vi "Chris_DAQ_100PSI.vi"() -> ()   [LabVIEW 2015]
uses:
  <vilib>/DAQmx/read.llb/DAQmx Read (Analog DBL 1Chan 1Samp).vi
  <vilib>/Instr/_visa.llb/VISA Configure Serial Port (Instr).vi
  <vilib>/DAQmx/create/channels.llb/DAQmx Create Channel (AI-Voltage-Basic).vi
  <vilib>/DAQmx/miscellaneous.llb/DAQmx Fill In Error Info.vi
panel:
  out "x/y":dbl
  in  "milliseconds to wait":u32
  out "Elapsed Time (s)":dbl
  out "time string":string
  in  "physical channels":tag
  out "Inlet Pressure":dbl format="%.1f"
  out "Average Flux":dbl(graph)
  out "Average Pressure":dbl(graph)
  in  "Rolling Average Length (Pressure)":u16=25
  out "Status:":bool caption="2017-05-22 4:50 PM"
  in  "Debug":bool=TRUE
  out "Aquired Data (Real Time)":cluster{"Scalar":dbl, "Filtered Volume":dbl}(graph)
  in  "Stop":bool
  out "Filtered Volume":dbl format="%.2g"
  in  "Save Path":path
  in  "Data Preview":i32(listbox)
  in  "Rolling Average Length (Flux)":u16=100
  in  "Membrane Area (sq. mm)":dbl
  in  "NI USB DAQ":tag="cDAQ2Mod1"
  in  "Filtrate Density":dbl=0.05
  in  "Flag":bool=TRUE
  in  "Precision Balance Port":refnum<visa-resource-name>="COM4"
  # "Liquid-Gated Membrane"
  # "Real-Time Data Acquisition System"
  # "Started:"
  # "Setup"
  # "COM Settings"
  # "Last Measurement:"
  # "Elapsed Time (s):"
  # "Measurement Settings"
  # "Last Updated: May 2017 • Chris Williams"
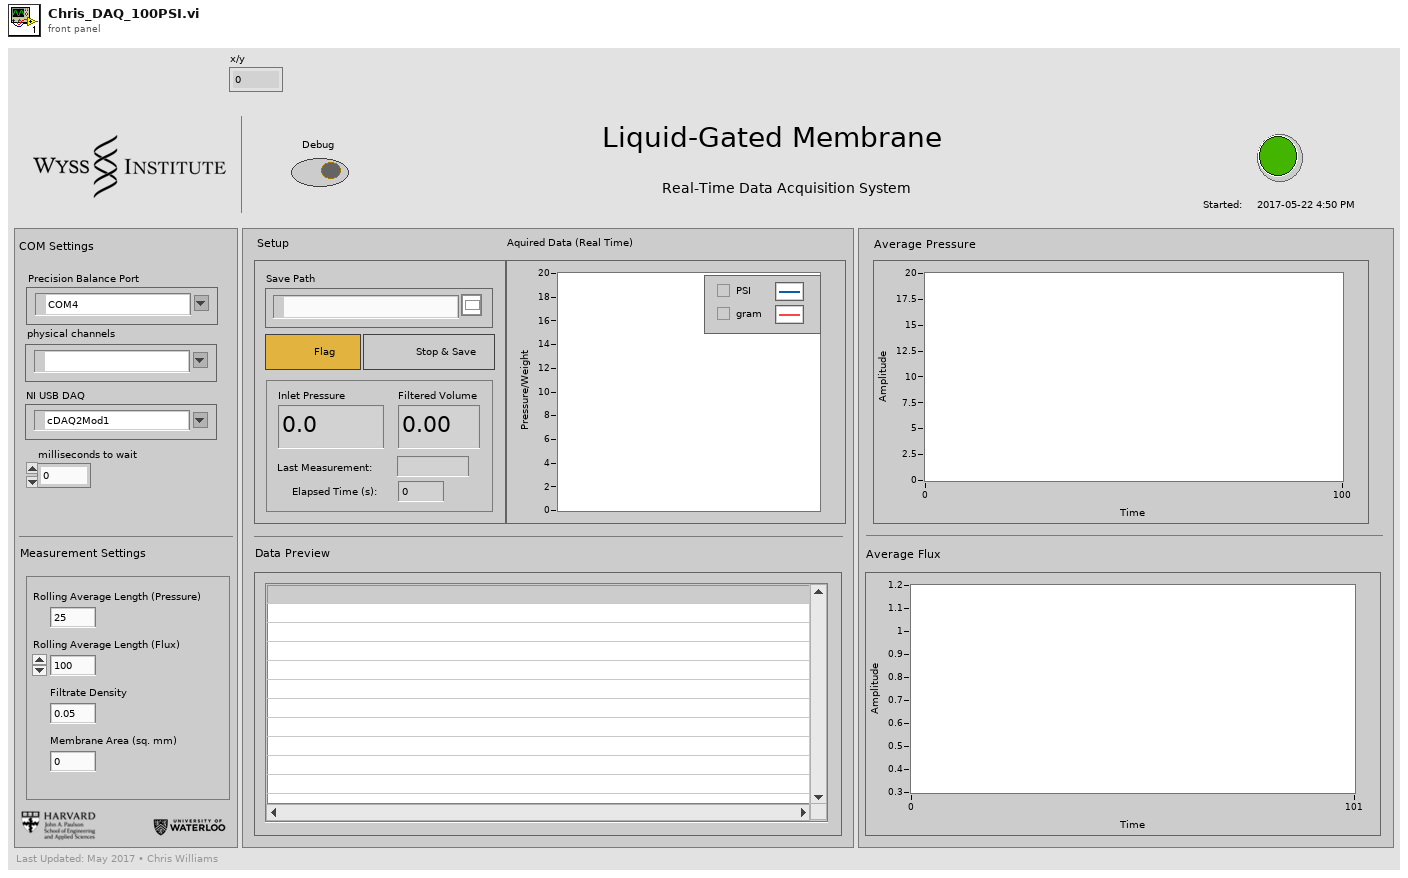
[diagram p1: front panel]
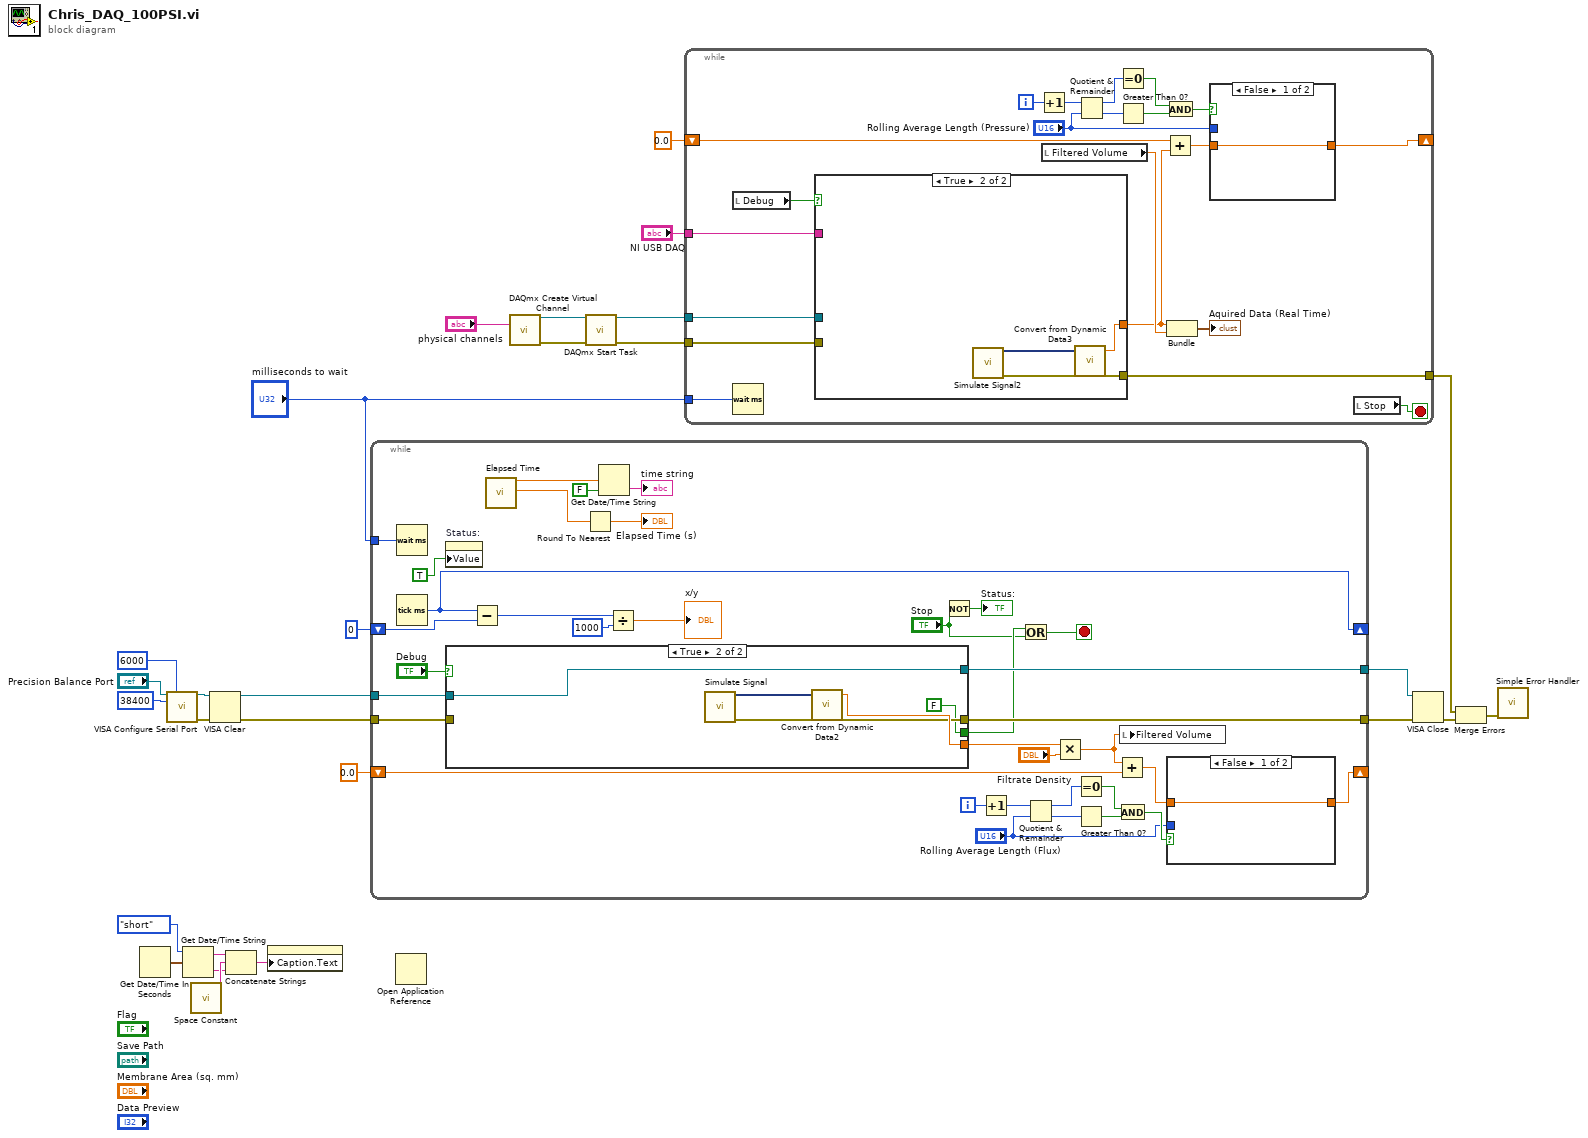
[diagram p0: block diagram]
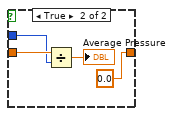
[diagram p2: hidden frame]
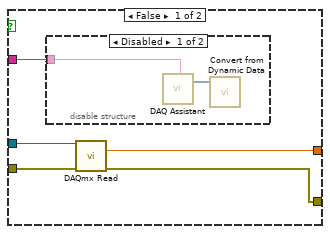
[diagram p3: hidden frame]
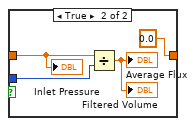
[diagram p5: hidden frame]
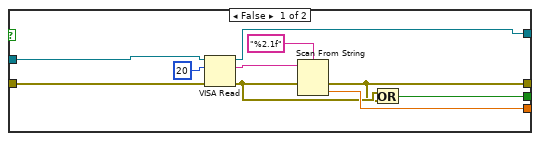
[diagram p6: hidden frame]
diagram:
  n1 = Get Date/Time In Seconds() -> (seconds since 1Jan1904=w8:timestamp)
  n2 = call-poly "VISA Configure Serial Port"("VISA resource name"="Precision Balance Port", "timeout (10sec)"=u32 6000, "baud rate (9600)"=u32 38400) -> ("VISA resource name out"=w24:refnum<visa-resource-name>, "error out"=w22:errorcluster)  [unwired: 11 in]
  n3 = Get Date/Time String(date format (0)=enum16{"short", "long", "abbreviated"}."short", seconds (now)=w8) -> (date string=w5:string, time string=w3:string)  [unwired: 1 in]
  n4 = call <vilib>:"Space Constant.vi"() -> ("String"=w6:string)
  n5 = VISA Clear(VISA resource name=w24, error in (no error)=w22) -> (VISA resource name out=w23:refnum<visa-resource-name>, error out=w21:errorcluster)
  n6 = Concatenate Strings(w5, w6, w3) -> (w4:string)
  n7 = property on="Status:" class="Bool (strict)"("Caption.Text"=w4) -> ()  [unwired: 2 in, 2 out]
  n8 = while {
    tunnel: w21 -> [w59]
    tunnel: [w60] -> w26
    tunnel: w23 -> [w61]
    tunnel: [w63] -> w25
    shift-right: [w45] -> _
    shift-left: 0.0 -> [w55]
    tunnel: "milliseconds to wait" -> [w38]
    shift-right: [w36] -> _
    shift-left: u32 0 ("millisecond timer value") -> [w37]
    i -> [w54]
    stop <- w32 stop-if-true
    n9 = Wait (ms)(milliseconds to wait=w38) -> ()  [unwired: 1 out]
    n10 = Tick Count (ms)() -> (millisecond timer value=w36:u32)
    n11 = property on="Status:" class="Bool (strict)"("Value"=TRUE ("Status:")) -> ()  [unwired: 2 in, 2 out]
    n12 = case shown="True" "Debug" {
      tunnel: [w78 w80] -> w63
      tunnel: [w75 w82] -> w44
      tunnel: w59 -> [w74 _]
      tunnel: w61 -> [w73 w80]
      tunnel: [w69 w81] -> w60
      tunnel: [w71 FALSE] -> w58
      frame False {
        n13 = VISA Read(VISA resource name=w73, byte count=u32 20, error in (no error)=w74) -> (VISA resource name out=w78:refnum<visa-resource-name>, read buffer=w77:string, error out=w70:errorcluster)  [unwired: 1 out]
        n14 = Scan From String(format string="%2.1f", input string=w77, error in=w70) -> (error out=w69:errorcluster, output 1=w75:dbl)  [unwired: 2 in, 2 out]
        n15 = Or(x=w70, y=w69) -> (x .or. y?=w71:bool)
      }
      frame True {
        n16 = call "Simulate Signal"() -> ("Triangle with Uniform Noise"=w83:dynamicdata, "error out"=w81:errorcluster)  [unwired: 14 in]
        n17 = call "Convert from Dynamic Data2"("Dynamic Data Type"=w83) -> ("Scalar"=w82:dbl)  [unwired: 3 in]
      }
    }
    n18 = Subtract(x=w36, y=w37) -> (x-y=w35:u32)
    n19 = call "Elapsed Time"() -> ("Present (s)"=w43:dbl, "Elapsed Time (s)"=w39:dbl)  [unwired: 12 in, 6 out]
    n20 = Round To Nearest(number=w39) -> (nearest integer value=→"Elapsed Time (s)":dbl)
    n21 = Get Date/Time String(seconds (now)=w43, want seconds? (F)=FALSE) -> (time string=→"time string":string)  [unwired: 1 in, 1 out]
    n22 = Divide(x=w35, y=u32 1000) -> (x/y=→"x/y":dbl)
    n23 = Not(x="Stop") -> (.not. x?=→"Status:":bool)
    n24 = Increment(x=w54) -> (x+1=w46:i32)
    n25 = Or(x=w58, y="Stop") -> (x .or. y?=w32:bool)
    n26 = Quotient & Remainder(x=w46, y="Rolling Average Length (Flux)") -> (x-y*floor(x/y)=w52:i32, floor(x/y)=w53:i32)
    n27 = Multiply(x=w44, y="Filtrate Density") -> (x*y=w56:dbl)
    n28 = Equal To 0?(x=w52) -> (x = 0?=w51:bool)
    n29 = Greater Than 0?(x=w53) -> (x > 0?=w50:bool)
    n30 = Add(x=w56, y=w55) -> (x+y=w48:dbl)
    n31 = And(x=w51, y=w50) -> (x .and. y?=w49:bool)
    n32 = local write "Filtered Volume"(w56) -> ()
    n33 = case shown="False" w49 {
      tunnel: w48 -> [w64 w65]
      tunnel: "Rolling Average Length (Flux)" -> [_ w68]
      tunnel: [w64 0.0 ("x+y")] -> w45
      frame False {
      }
      frame True {
        n34 = Divide(x=w65, y=w68) -> (x/y=→"Average Flux" →"Filtered Volume":dbl)
        "Inlet Pressure" <- w65
      }
    }
  }
  n35 = Open Application Reference() -> ()  [unwired: 4 in, 2 out]
  n36 = call-poly <vilib>:"DAQmx Create Virtual Channel.vi"("physical channels"="physical channels") -> ("task out"=w12:refnum<k21>, "error out"=w11:errorcluster)  [unwired: 13 in]
  n37 = call <vilib>:"DAQmx Start Task.vi"("task/channels in"=w12, "error in"=w11) -> ("task out"=w10:refnum<k21>, "error out"=w9:errorcluster)  [unwired: 12 in]
  n38 = while {
    tunnel: "NI USB DAQ" -> [w104]
    tunnel: [w103] -> w19
    shift-right: [w95] -> _
    shift-left: 0.0 ("Scalar") -> [w97]
    tunnel: w10 -> [w86]
    tunnel: w9 -> [w85]
    tunnel: "milliseconds to wait" -> [w84]
    i -> [w94]
    stop <- w102 stop-if-true
    n39 = local read "Debug"() -> (w99:bool)
    n40 = Wait (ms)(milliseconds to wait=w84) -> ()  [unwired: 1 out]
    n41 = case shown="True" w99 {
      tunnel: w104 -> [w114 _]
      tunnel: [w110 w119] -> w103
      tunnel: [w111 w117] -> w98
      tunnel: w86 -> [w113 _]
      tunnel: w85 -> [w112 _]
      frame False {
        n42 = disable-structure shown="Disabled" {
          disable-tunnel: w114 -> [w116 _]
          frame Disabled {
            n43 = call "DAQ Assistant"("device name"=w116) -> ("data"=w115:dynamicdata)  [unwired: 15 in, 3 out]
            n44 = call "Convert from Dynamic Data"("Dynamic Data Type"=w115) -> ()  [unwired: 3 in, 1 out]
          }
          frame Enabled {
          }
        }
        n45 = call-poly <vilib>:"DAQmx Read.vi"("task/channels in"=w113, "error in"=w112) -> ("data"=w111:dbl, "error out"=w110:errorcluster)  [unwired: 11 in, 1 out]
      }
      frame True {
        n46 = call "Simulate Signal2"() -> ("Sine with Uniform Noise"=w118:dynamicdata, "error out"=w119:errorcluster)  [unwired: 14 in]
        n47 = call "Convert from Dynamic Data3"("Dynamic Data Type"=w118) -> ("Scalar"=w117:dbl)  [unwired: 3 in]
      }
    }
    n48 = Increment(x=w94) -> (x+1=w93:i32)
    n49 = local read "Filtered Volume"() -> (w101:dbl)
    n50 = Quotient & Remainder(x=w93, y="Rolling Average Length (Pressure)") -> (x-y*floor(x/y)=w92:i32, floor(x/y)=w91:i32)
    n51 = Equal To 0?(x=w92) -> (x = 0?=w90:bool)
    n52 = Greater Than 0?(x=w91) -> (x > 0?=w89:bool)
    n53 = Add(x=w97, y=w98) -> (x+y=w96:dbl)
    n54 = And(x=w90, y=w89) -> (x .and. y?=w88:bool)
    n55 = Bundle("Scalar"=w98, "Filtered Volume"=w101) -> (→"Aquired Data (Real Time)":cluster{"Scalar":dbl, "Filtered Volume":dbl})  [unwired: 1 in]
    n56 = case shown="False" w88 {
      tunnel: w96 -> [w105 w109]
      tunnel: [w105 0.0] -> w95
      tunnel: "Rolling Average Length (Pressure)" -> [_ w108]
      frame False {
      }
      frame True {
        n57 = Divide(x=w109, y=w108) -> (x/y=→"Average Pressure":dbl)
      }
    }
    n58 = local read "Stop"() -> (w102:bool)
  }
  n59 = VISA Close(VISA resource name=w25, error in (no error)=w26) -> (error out=w18:errorcluster)
  n60 = Merge Errors(w19, w18) -> (w17:errorcluster)
  n61 = call <vilib>:"Simple Error Handler.vi"("error in (no error)"=w17) -> ()  [unwired: 4 in, 5 out]
